vi "Lobatto Weights (4&7 order).vi"(10 "lower limit":dbl, 11 "upper limit":dbl) -> (2 "Weights (7-Order)":dbl[](array[numeric]), 3 "Weights (4-Order)":dbl[](array[numeric]))   [LabVIEW 2018, in "NI_AALPro.lvlib"]
uses:
  NI_AALPro.lvlib
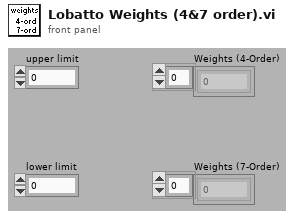
[diagram p1: front panel]
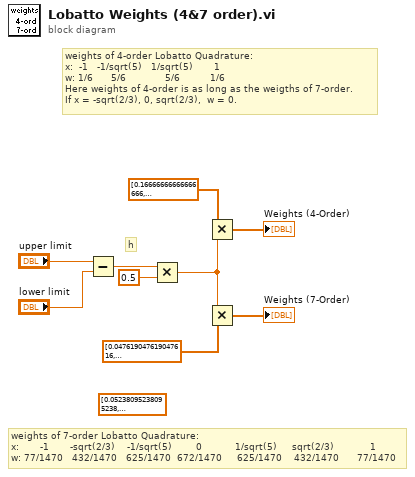
[diagram p0: block diagram]
diagram:
  (unwired) dbl[] [0.05238095238095238, 0.2938775510204082, 0.42517006802721086, 0.45714285714285713, 0.42517006802721086, 0.2938775510204082, 0.05238095238095238] ("x/y 2")
  # "weights of 7-order Lobatto Quadrature:\nx:       -1       -sqrt(2/3)    -1/sqrt(5)        0           1/sqrt(5)     sqrt(2/3)            1\nw: 77/1470   432/1470   625/1470  672/1470     625/1470    432/1470      77/1470"
  # "weights of 4-order Lobatto Quadrature:\nx:  -1   -1/sqrt(5)   1/sqrt(5)       1\nw: 1/6      5/6             5/6          1/6\nHere weights of 4-order is as long as the weigths of 7-order.\nIf x = -sqrt(2/3), 0, sqrt(2/3),  w = 0."
  # "h"
  n1 = Subtract(x="upper limit", y="lower limit") -> (x-y=w5:dbl)
  n2 = Multiply(x=w5, y=0.5) -> (x*y=w2:dbl)
  n3 = Multiply(x=dbl[] [0.16666666666666666, 0.8333333333333334, 0.8333333333333334, 0.16666666666666666] ("x/y"), y=w2) -> (x*y=→"Weights (4-Order)":dbl[])
  n4 = Multiply(x=w2, y=dbl[] [0.047619047619047616, 0.2768260473615695, 0.431745381209862, 0.4876190476190476, 0.431745381209862, 0.2768260473615695, 0.047619047619047616] ("appended array 2")) -> (x*y=→"Weights (7-Order)":dbl[])
